vi "Get Current Date.vi"() -> (6 "Date String":string)   [LabVIEW 2022 SP3]
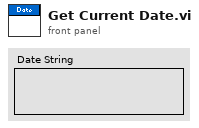
[diagram p1: front panel]
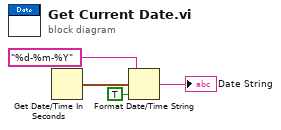
[diagram p0: block diagram]
diagram:
  n1 = Get Date/Time In Seconds() -> (seconds since 1Jan1904=w1:timestamp)
  n2 = Format Date/Time String(time format string (%c)="%d-%m-%Y", seconds (now)=w1, UTC format=TRUE) -> (date/time string=→"Date String":string)
